vi "simple calculator.vi"() -> ()   [LabVIEW 2019]
panel:
  in  "stop":bool
  out "Display":string
  in  "Buttons":T1
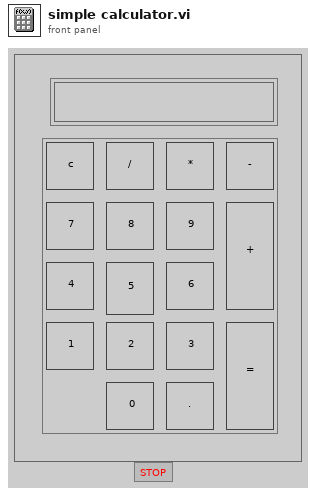
[diagram p1: front panel]
types:
  T1 = cluster{"clear":bool, "div":bool, "mul":bool, "sub":bool, "seven":bool, "eight":bool, "nine":bool, "four":bool, "five":bool, "six":bool, "one":bool, "two":bool, "three":bool, "zero":bool, "dot":bool, "sum":bool, "equal to":bool}
  T2 = enum16{"no function", "sum", "sub", "mul", "div"}
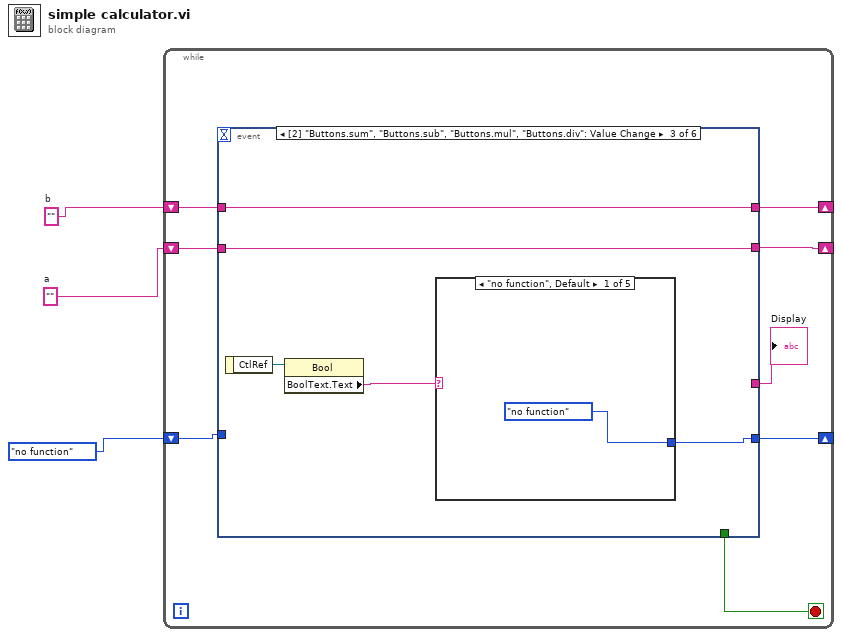
[diagram p0: block diagram]
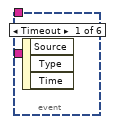
[diagram p2: hidden frame]
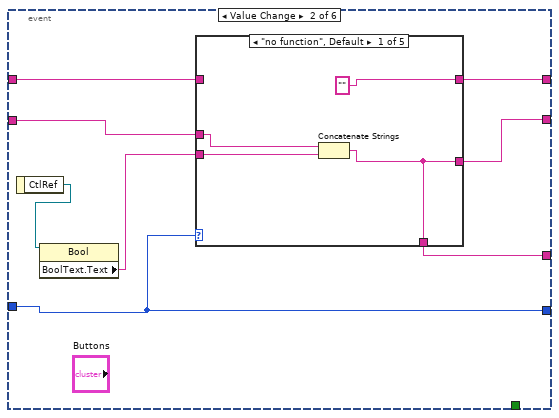
[diagram p3: hidden frame]
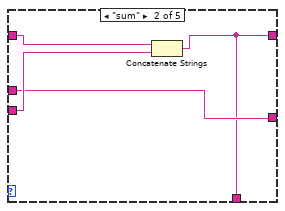
[diagram p4: hidden frame]
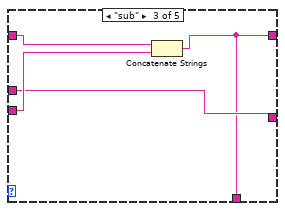
[diagram p5: hidden frame]
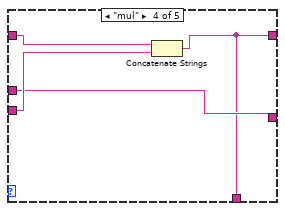
[diagram p6: hidden frame]
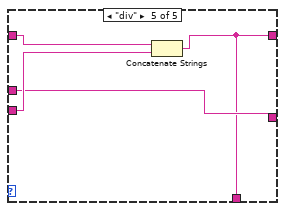
[diagram p7: hidden frame]
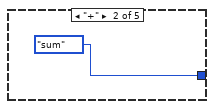
[diagram p8: hidden frame]
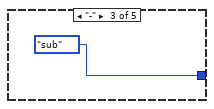
[diagram p9: hidden frame]
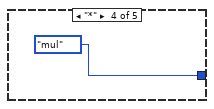
[diagram p10: hidden frame]
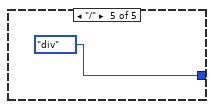
[diagram p11: hidden frame]
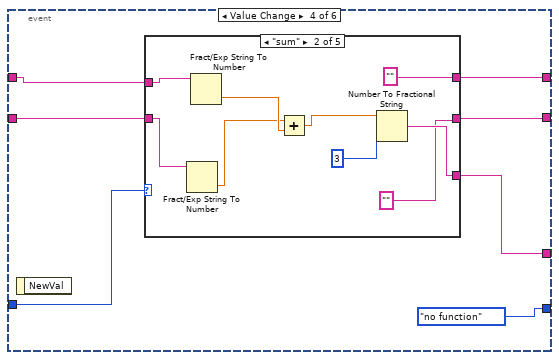
[diagram p12: hidden frame]
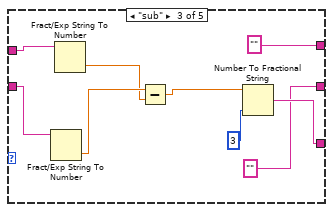
[diagram p14: hidden frame]
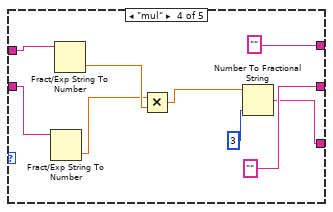
[diagram p15: hidden frame]
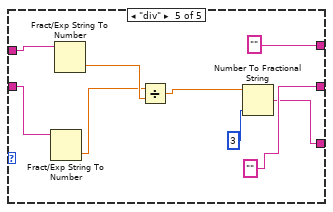
[diagram p16: hidden frame]
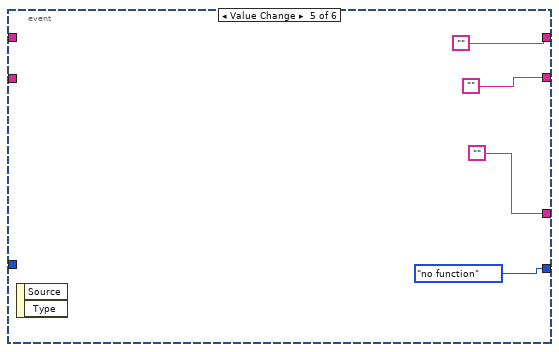
[diagram p17: hidden frame]
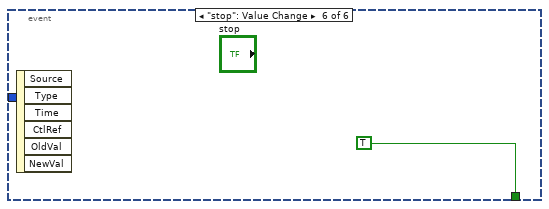
[diagram p18: hidden frame]
diagram:
  w2 = ""  # a
  w1 = ""  # b
  n1 = while {
    shift-right: [w7] -> _
    shift-left: w1 -> [w8]
    shift-right: [w6] -> _
    shift-left: w2 -> [w9]
    shift-right: [w10] -> _
    shift-left: T2."no function" -> [w11]
    stop <- w4 stop-if-true
    n2 = event shown="[2] \"Buttons.sum\", \"Buttons.sub\", \"Buttons.mul\", \"Buttons.div\": Value Change" {
      selector: _ -> [_ _ _ _ _ _]
      dyn-events: _ -> [_ _ _ _ _ _]
      timeout: _ -> [_ _ _ _ _ _]
      tunnel: w11 -> [_ w19 _ w56 _ _]
      tunnel: [_ w19 w42 T2."no function" T2."no function" _] -> w10
      tunnel: w9 -> [_ w18 w41 w54 _ _]
      tunnel: w8 -> [_ w15 w40 w55 _ _]
      tunnel: [_ w14 w40 w53 "" _] -> w7
      tunnel: [_ w13 w41 w52 "" _] -> w6
      tunnel: [_ w12 _ w50 "" _] -> w5
      tunnel: [_ _ _ _ _ TRUE] -> w4
      event Timeout {
        n3 = event-data() -> ()  [unwired: 1 in, 3 out]
      }
      event "Buttons.seven", "Buttons.eight", "Buttons.nine", "Buttons.four", "Buttons.five", "Buttons.six", "Buttons.one", "Buttons.two", "Buttons.three", "Buttons.zero", "Buttons.dot": Value Change {
        n4 = event-data() -> ("CtlRef"=w17:refnum<vi>)  [unwired: 1 in]
        n5 = property class="Bool"(reference=w17) -> ("BoolText.Text"=w16:string)  [unwired: 1 in, 2 out]
        n6 = case shown="\"no function\", Default" w19 {
          tunnel: w18 -> [w23 w25 w29 w33 w37]
          tunnel: w16 -> [w22 w27 w31 w35 w39]
          tunnel: w15 -> [_ w26 w30 w34 w38]
          tunnel: ["" w24 w28 w32 w36] -> w14
          tunnel: [w20 w25 w29 w33 w37] -> w13
          tunnel: [w20 w24 w28 w32 w36] -> w12
          frame "no function", Default {
            n7 = Concatenate Strings(w23, w22) -> (w20:string)
          }
          frame "sum" {
            n8 = Concatenate Strings(w26, w27) -> (w24:string)
          }
          frame "sub" {
            n9 = Concatenate Strings(w30, w31) -> (w28:string)
          }
          frame "mul" {
            n10 = Concatenate Strings(w34, w35) -> (w32:string)
          }
          frame "div" {
            n11 = Concatenate Strings(w38, w39) -> (w36:string)
          }
        }
      }
      event "Buttons.sum", "Buttons.sub", "Buttons.mul", "Buttons.div": Value Change {
        n12 = event-data() -> ("CtlRef"=w44:refnum<vi>)  [unwired: 1 in]
        n13 = property class="Bool"(reference=w44) -> ("BoolText.Text"=w43:string)  [unwired: 1 in, 2 out]
        n14 = case shown="\"no function\", Default" w43 {
          tunnel: [T2."no function" T2."sum" T2."sub" T2."mul" T2."div"] -> w42
          frame "no function", Default {
          }
          frame "+" {
          }
          frame "-" {
          }
          frame "*" {
          }
          frame "/" {
          }
        }
      }
      event "Buttons.equal to": Value Change {
        n15 = event-data() -> ()  [unwired: 1 in, 1 out]
        n16 = case shown="\"sum\"" w56 {
          tunnel: w55 -> [w58 w65 w74 w83 w92]
          tunnel: w54 -> [w57 w64 w73 w82 w91]
          tunnel: [w58 "" ("b") "" ("b") "" ("b") "" ("b")] -> w53
          tunnel: [w57 "" ("b") "" ("b") "" ("b") "" ("b")] -> w52
          tunnel: [w57 w60 w69 w77 w86] -> w50
          frame "no function", Default {
          }
          frame "sum" {
            n17 = Fract/Exp String To Number(string=w64) -> (number=w62:dbl)  [unwired: 3 in, 1 out]
            n18 = Fract/Exp String To Number(string=w65) -> (number=w63:dbl)  [unwired: 3 in, 1 out]
            n19 = Add(x=w62, y=w63) -> (x+y=w61:dbl)
            n20 = Number To Fractional String(number=w61, precision (6)=i16 3) -> (F-format string=w60:string)  [unwired: 2 in]
          }
          frame "sub" {
            n21 = Fract/Exp String To Number(string=w73) -> (number=w72:dbl)  [unwired: 3 in, 1 out]
            n22 = Fract/Exp String To Number(string=w74) -> (number=w71:dbl)  [unwired: 3 in, 1 out]
            n23 = Subtract(x=w72, y=w71) -> (x-y=w70:dbl)
            n24 = Number To Fractional String(number=w70, precision (6)=i16 3) -> (F-format string=w69:string)  [unwired: 2 in]
          }
          frame "mul" {
            n25 = Fract/Exp String To Number(string=w82) -> (number=w80:dbl)  [unwired: 3 in, 1 out]
            n26 = Fract/Exp String To Number(string=w83) -> (number=w81:dbl)  [unwired: 3 in, 1 out]
            n27 = Multiply(x=w80, y=w81) -> (x*y=w79:dbl)
            n28 = Number To Fractional String(number=w79, precision (6)=i16 3) -> (F-format string=w77:string)  [unwired: 2 in]
          }
          frame "div" {
            n29 = Fract/Exp String To Number(string=w91) -> (number=w89:dbl)  [unwired: 3 in, 1 out]
            n30 = Fract/Exp String To Number(string=w92) -> (number=w90:dbl)  [unwired: 3 in, 1 out]
            n31 = Divide(x=w89, y=w90) -> (x/y=w88:dbl)
            n32 = Number To Fractional String(number=w88, precision (6)=i16 3) -> (F-format string=w86:string)  [unwired: 2 in]
          }
        }
      }
      event "Buttons.clear": Value Change {
        n33 = event-data() -> ()  [unwired: 1 in, 2 out]
      }
      event "stop": Value Change {
        n34 = event-data() -> ()  [unwired: 1 in, 6 out]
      }
    }
    "Display" <- w5
  }
